vi "The Game.vi"() -> ()   [LabVIEW 2023]
panel:
  out "Start seconds":dbl
  out "Seconds":i16
  out "Minutes":i16
  out "Hours":i16
  out "Response window":string="Input a guess into the input window.\nHave a guess!"
  in  "Number \nof \ncorrect \nguesses":dbl
  in  "Input window":string
  in  "stop":bool
  out "Table Control":string[][](table)=[["1", ""], ["2", ""], ["3", ""], ["4", ""], ["5", ""], ["6", ""], ["7", ""], ["8", ""], ["9", ""], ["", "Noe"]]
  # "Pokemon Quiz Game!"
  # "Guess the names of starter Pokemon, from the Kanto region \nusing the input window and check how quickly you can do \nit! Good Luck!"
  # "Time used:"
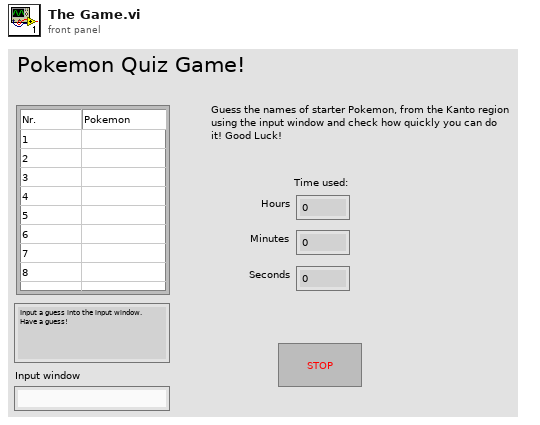
[diagram p1: front panel]
types:
  T1 = enum8{"Enabled", "Disabled", "Disabled and Grayed Out"}
  T2 = typedef "eventvkey.ctl" = enum16{"ASCII", "Enter", "Return", "Shift", "Ctrl", "Alt", "Cmd", "Opt", "Caps", "NumLock", "Clear", "Break", "Up", "Down", "Left", "Right", "Insert", "Delete", "Home", "End", "PageUp", "PageDown", "Escape", "Help", "Pause", "ScrollLock", "F1", "F2", "F3", "F4", "F5", "F6", "F7", "F8", "F9", "F10", "F11", "F12", "F13", "F14", "F15", "F16", "F17", "F18", "F19", "F20", "F21", "F22", "F23", "F24", "Play", "VolumeUp", "VolumeDown", "Mute", "Two Byte Char"}
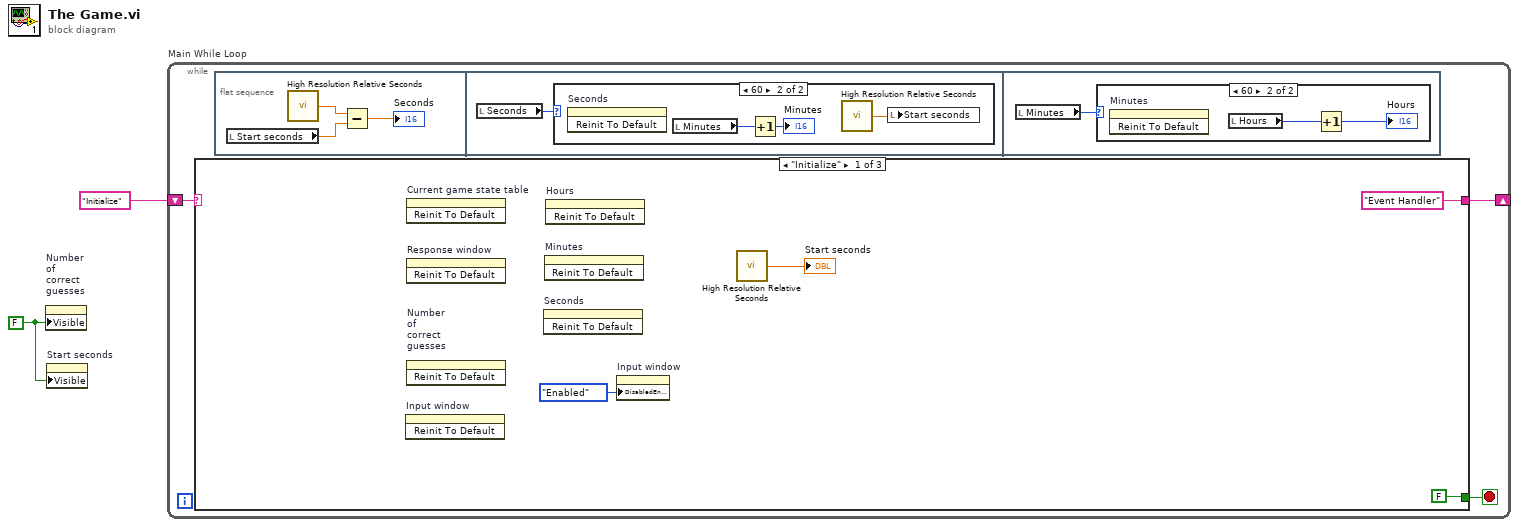
[diagram p0: block diagram]
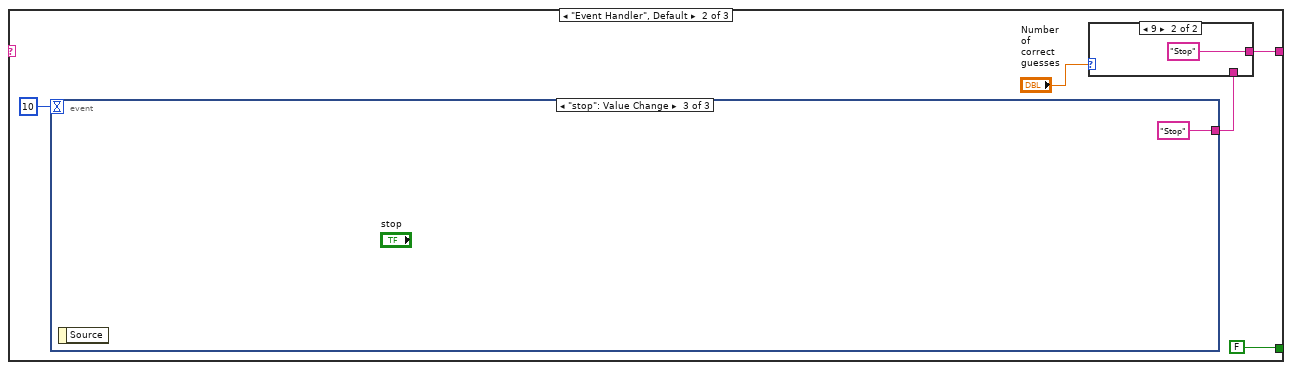
[diagram p4: hidden frame]
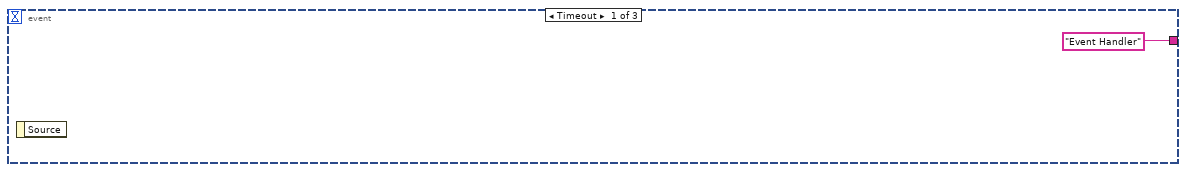
[diagram p6: hidden frame]
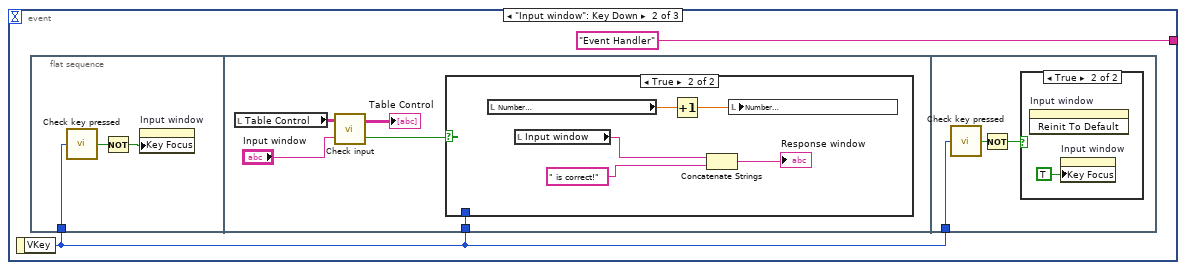
[diagram p7: hidden frame]
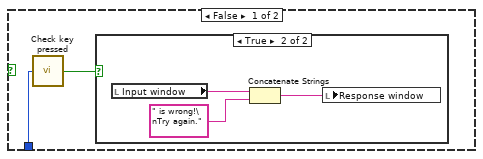
[diagram p8: hidden frame]
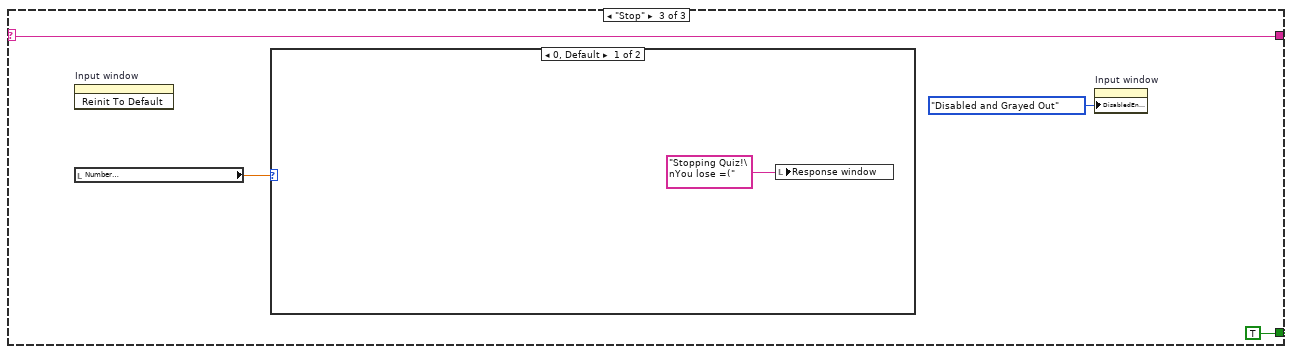
[diagram p11: hidden frame]
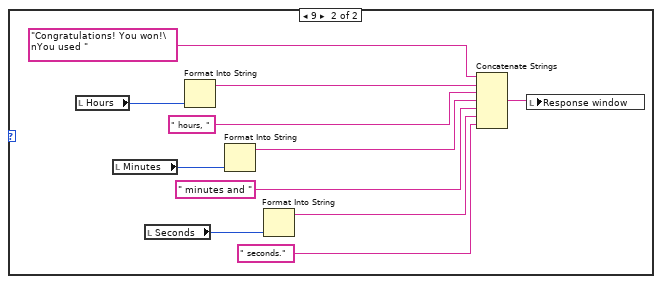
[diagram p12: hidden frame]
diagram:
  w1 = FALSE ("Visible")
  n1 = property on="Number \nof \ncorrect \nguesses" class="DigNum (strict)"("Visible"=w1) -> ()  [unwired: 2 in, 2 out]
  n2 = property on="Start seconds" class="DigNum (strict)"("Visible"=w1) -> ()  [unwired: 2 in, 2 out]
  n3 = while "Main While Loop" {
    shift-right: [w4] -> _
    shift-left: "Initialize" -> [w5]
    stop <- w3 stop-if-true
    n4 = case shown="\"Initialize\"" w5 {
      selector: w5 -> [_ _ w56]
      tunnel: ["Event Handler" w20 w56] -> w4
      tunnel: [FALSE FALSE TRUE] -> w3
      frame "Initialize" {
        n5 = invoke on="Input window" class="Str" method="Reinit To Default"() -> ()  [unwired: 3 in, 3 out]
        n6 = invoke on="Current game state table" class="Tbl (strict)" method="Reinit To Default"() -> ()  [unwired: 3 in, 3 out]
        n7 = invoke on="Response window" class="Str" method="Reinit To Default"() -> ()  [unwired: 3 in, 3 out]
        n8 = invoke on="Number \nof \ncorrect \nguesses" class="DigNum (strict)" method="Reinit To Default"() -> ()  [unwired: 3 in, 3 out]
        n9 = invoke on="Seconds" class="DigNum (strict)" method="Reinit To Default"() -> ()  [unwired: 3 in, 3 out]
        n10 = invoke on="Minutes" class="DigNum (strict)" method="Reinit To Default"() -> ()  [unwired: 3 in, 3 out]
        n11 = invoke on="Hours" class="DigNum (strict)" method="Reinit To Default"() -> ()  [unwired: 3 in, 3 out]
        n12 = property on="Input window" class="Str"("DisabledEnum"=T1."Enabled" ("Disabled")) -> ()  [unwired: 2 in, 2 out]
        n13 = call <vilib>:"High Resolution Relative Seconds.vi"() -> ("relative seconds"=→"Start seconds":dbl)
      }
      frame "Event Handler", Default {
        n14 = event shown="[2] \"stop\": Value Change" {
          selector: _ -> [_ _ _]
          dyn-events: _ -> [_ _ _]
          timeout: 10 -> [_ _ _]
          tunnel: ["Event Handler" "Event Handler" "Stop"] -> w22
          event Timeout {
            n15 = event-data() -> ()  [unwired: 1 in, 1 out]
          }
          event "Input window": Key Down {
            n16 = event-data() -> ("VKey"=w28:T2)  [unwired: 1 in]
            n17 = flat-sequence {
              tunnel: w28 -> [w32]
              tunnel: w28 -> [w33]
              tunnel: w28 -> [w50]
              frame #0 {
                n18 = call "Check key pressed.vi"("Key pressed"=w32) -> ("Enter was pressed?"=w31:bool)
                n19 = Not(x=w31) -> (.not. x?=w30:bool)
                n20 = property on="Input window" class="Str"("Key Focus"=w30) -> ()  [unwired: 2 in, 2 out]
              }
              frame #1 {
                n21 = local read "Table Control"() -> (w36:string[][])
                n22 = call "Check input.vi"("String to check for"="Input window", "Old table to replace"=w36) -> ("Guess is correct?"=w35:bool, "Output table"=→"Table Control":string[][])
                n23 = case shown="True" w35 {
                  tunnel: w33 -> [w39 _]
                  frame False {
                    n24 = call "Check key pressed.vi"("Key pressed"=w39) -> ("Enter was pressed?"=w38:bool)
                    n25 = case shown="True" w38 {
                      frame False {
                      }
                      frame True {
                        n26 = local read "Input window"() -> (w40:string)
                        n27 = Concatenate Strings "Concatenate Strings"(w40, " is wrong!\nTry again." ("Response window")) -> (w41:string)
                        n28 = local write "Response window"(w41) -> ()
                      }
                    }
                  }
                  frame True {
                    n29 = local read "Number \nof \ncorrect \nguesses"() -> (w46:dbl)
                    n30 = local read "Input window"() -> (w44:string)
                    n31 = Increment(x=w46) -> (x+1=w47:dbl)
                    n32 = Concatenate Strings "Concatenate Strings"(w44, " is correct!" ("Response window")) -> (→"Response window":string)
                    n33 = local write "Number \nof \ncorrect \nguesses"(w47) -> ()
                  }
                }
              }
              frame #2 {
                n34 = call "Check key pressed.vi"("Key pressed"=w50) -> ("Enter was pressed?"=w49:bool)
                n35 = Not(x=w49) -> (.not. x?=w48:bool)
                n36 = case shown="True" w48 {
                  frame False {
                  }
                  frame True {
                    n37 = invoke on="Input window" class="Str" method="Reinit To Default"() -> ()  [unwired: 3 in, 3 out]
                    n38 = property on="Input window" class="Str"("Key Focus"=TRUE) -> ()  [unwired: 2 in, 2 out]
                  }
                }
              }
            }
          }
          event "stop": Value Change {
            n39 = event-data() -> ()  [unwired: 1 in, 1 out]
          }
        }
        n40 = case shown="9" "Number \nof \ncorrect \nguesses" {
          tunnel: [w25 "Stop"] -> w20
          tunnel: w22 -> [w25 _]
          frame 0, Default {
          }
          frame 9 {
          }
        }
      }
      frame "Stop" {
        n41 = invoke on="Input window" class="Str" method="Reinit To Default"() -> ()  [unwired: 3 in, 3 out]
        n42 = local read "Number \nof \ncorrect \nguesses"() -> (w53:dbl)
        n43 = case shown="0, Default" w53 {
          frame 0, Default {
            n44 = local write "Response window"("Stopping Quiz!\nYou lose =(" ("Response window")) -> ()
          }
          frame 9 {
            n45 = local read "Hours"() -> (w67:i16)
            n46 = local read "Minutes"() -> (w64:i16)
            n47 = local read "Seconds"() -> (w63:i16)
            n48 = Format Into String "Format Into String"(w67) -> (resulting string=w66:string)  [unwired: 3 in, 1 out]
            n49 = Format Into String "Format Into String"(w64) -> (resulting string=w62:string)  [unwired: 3 in, 1 out]
            n50 = Format Into String "Format Into String"(w63) -> (resulting string=w61:string)  [unwired: 3 in, 1 out]
            n51 = Concatenate Strings "Concatenate Strings"("Congratulations! You won!\nYou used " ("Response window"), w66, " hours, " ("string"), w62, " minutes and " ("string"), w61, " seconds." ("string")) -> (w58:string)
            n52 = local write "Response window"(w58) -> ()
          }
        }
        n53 = property on="Input window" class="Str"("DisabledEnum"=T1."Disabled and Grayed Out" ("Disabled")) -> ()  [unwired: 2 in, 2 out]
      }
    }
    n54 = flat-sequence {
      frame #0 {
        n55 = local read "Start seconds"() -> (w6:dbl)
        n56 = call <vilib>:"High Resolution Relative Seconds.vi"() -> ("relative seconds"=w7:dbl)
        n57 = Subtract(x=w7, y=w6) -> (x-y=→"Seconds":dbl)
      }
      frame #1 {
        n58 = local read "Seconds"() -> (w9:i16)
        n59 = case shown="60" w9 {
          frame 0, Default {
          }
          frame 60 {
            n60 = invoke on="Seconds" class="DigNum (strict)" method="Reinit To Default"() -> ()  [unwired: 3 in, 3 out]
            n61 = local read "Minutes"() -> (w11:i16)
            n62 = Increment(x=w11) -> (x+1=→"Minutes":i16)
            n63 = call <vilib>:"High Resolution Relative Seconds.vi"() -> ("relative seconds"=w10:dbl)
            n64 = local write "Start seconds"(w10) -> ()
          }
        }
      }
      frame #2 {
        n65 = local read "Minutes"() -> (w13:i16)
        n66 = case shown="60" w13 {
          frame 0, Default {
          }
          frame 60 {
            n67 = invoke on="Minutes" class="DigNum (strict)" method="Reinit To Default"() -> ()  [unwired: 3 in, 3 out]
            n68 = local read "Hours"() -> (w15:i16)
            n69 = Increment(x=w15) -> (x+1=→"Hours":i16)
          }
        }
      }
    }
  }
